vi "Problem1.2.vi"() -> ()   [LabVIEW 2018]
panel:
  out "(A AND B) XOR (A XOR B)":bool
  in  "?":bool
  in  "B":bool
  out "Not B":bool
  out "Not A":bool
  out "XOR":bool
  out "Or":bool
  out "And":bool
  in  "A":bool
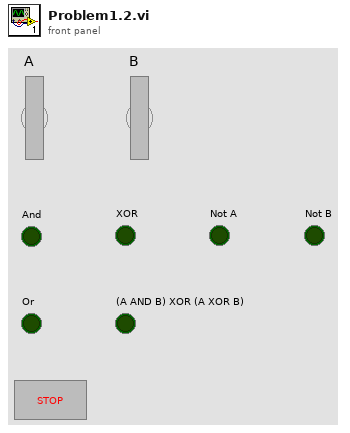
[diagram p1: front panel]
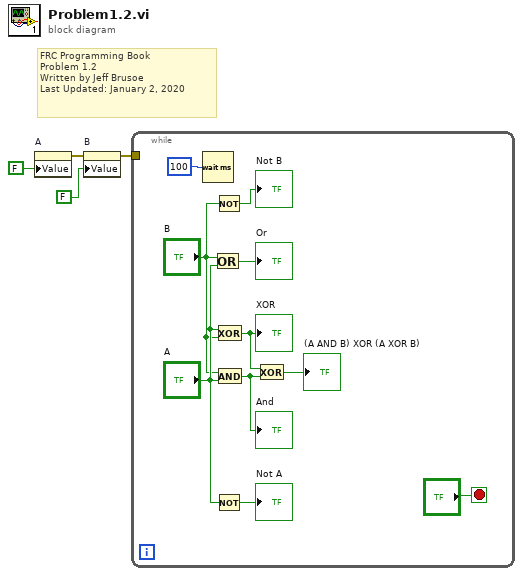
[diagram p0: block diagram]
diagram:
  # "FRC Programming Book\nProblem 1.2\nWritten by Jeff Brusoe\nLast Updated: January 2, 2020"
  n1 = property on="A" class="Bool (strict)"("Value"=FALSE ("A")) -> (error out=w2:errorcluster)  [unwired: 2 in, 1 out]
  n2 = property on="B" class="Bool (strict)"(error in=w2, "Value"=FALSE ("B")) -> (error out=w1:errorcluster)  [unwired: 1 in, 1 out]
  n3 = while {
    tunnel: w1 -> [_]
    stop <- "?" stop-if-true
    n4 = Wait (ms)(milliseconds to wait=u32 100) -> ()  [unwired: 1 out]
    n5 = Or(x="B", y="A") -> (x .or. y?=→"Or":bool)
    n6 = Not(x="B") -> (.not. x?=→"Not B":bool)
    n7 = Not(x="A") -> (.not. x?=→"Not A":bool)
    n8 = Exclusive Or(1:"B", 2:"A") -> (0:w5:bool)
    "XOR" <- w5
    n9 = And(x="B", y="A") -> (x .and. y?=w6:bool)
    "And" <- w6
    n10 = Exclusive Or(1:w6, 2:w5) -> (0:→"(A AND B) XOR (A XOR B)":bool)
  }
